vi "ProjectOpenReferences.vi"(0 "Project File Path":path, 5 "Gateway IP Address (\"\": localhost)":string, 11 "error in (no error)":errorcluster, 12 "Username":string, 13 "Password":string) -> (4 "Project File Path out":path, 6 "Gateway IP Address out":string, 15 "error out":errorcluster)   [LabVIEW 2020, in "ni-veristand-steps-runtime-lib.lvlib"]
uses:
  ni-veristand-steps-runtime-lib.lvlib
  controls/VeriStand dotNet References.ctl
  <vilib>/NI VeriStand/Execution/ModelManager/ModelManagerAPI.ctl
  <vilib>/NI VeriStand/Execution/AlarmManager/AlarmManagerAPI.ctl
  <vilib>/NI VeriStand/Execution/ChannelFaultManager/ChannelFaultAPI.ctl
  <vilib>/NI VeriStand/Execution/Workspace/WorkspaceAPI.ctl
  <vilib>/NI VeriStand/Execution/Project/Project Ref.ctl
  <vilib>/NI VeriStand/Execution/Workspace/NI_VS Workspace ExecutionAPI.lvlib
  <vilib>/NI VeriStand/Execution/ChannelFaultManager/NI_VS ChannelFault ExecutionAPI.lvlib
  <vilib>/NI VeriStand/Execution/ModelManager/NI_VS ModelManager ExecutionAPI.lvlib
  NationalInstruments.VeriStand.ClientAPI
  <vilib>/NI VeriStand/Execution/Project/NI_VS Project ExecutionAPI.lvlib
  <vilib>/NI VeriStand/Execution/AlarmManager/NI_VS AlarmManager ExecutionAPI.lvlib
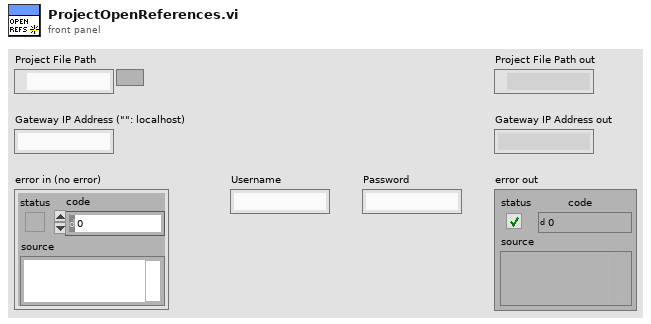
[diagram p1: front panel]
types:
  T1 = typedef "ni-veristand-steps-runtime-lib.lvlib/VeriStand dotNet References.ctl" = cluster{"ModelManager":T2, "AlarmManager":T3, "ChannelFault":T4, "WorkspaceManager":T5, "Project Ref":T6}
  T2 = typedef "NI_VS ModelManager ExecutionAPI.lvlib/ModelManagerAPI.ctl" = refnum<k24>
  T3 = typedef "NI_VS AlarmManager ExecutionAPI.lvlib/AlarmManagerAPI.ctl" = refnum<k24>
  T4 = typedef "NI_VS ChannelFault ExecutionAPI.lvlib/ChannelFaultAPI.ctl" = refnum<k24>
  T5 = typedef "NI_VS Workspace ExecutionAPI.lvlib/WorkspaceAPI.ctl" = refnum<k24>
  T6 = typedef "NI_VS Project ExecutionAPI.lvlib/Project Ref.ctl" = refnum<k24>
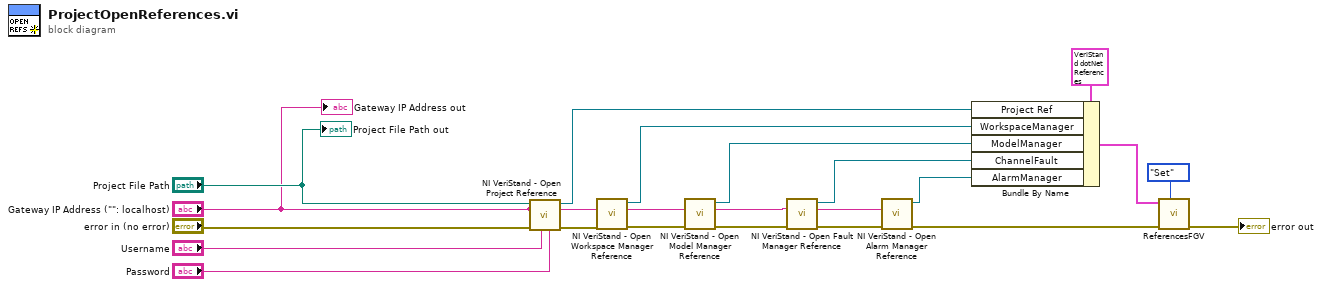
[diagram p0: block diagram]
diagram:
  n1 = call <vilib>:"NI VeriStand - Open Project Reference.vi"("Password"="Password", "Username"="Username", "error in (no error)"="error in (no error)", "Gateway IP Address (\"\": localhost)"="Gateway IP Address (\"\": localhost)", "Project File Path"="Project File Path") -> ("error out"=w6:errorcluster, "Project Ref"=w5:T6)  [unwired: 5 in]
  n2 = call <vilib>:"NI VeriStand - Open Workspace Manager Reference.vi"("error in (no error)"=w6, "Gateway IP Address (\"\": localhost)"="Gateway IP Address (\"\": localhost)") -> ("error out"=w19:errorcluster, "WorkspaceManager"=w12:T5)  [unwired: 8 in]
  n3 = call <vilib>:"NI VeriStand - Open Model Manager Reference.vi"("error in (no error)"=w19, "Gateway IP Address (\"\": localhost)"="Gateway IP Address (\"\": localhost)") -> ("error out"=w18:errorcluster, "ModelManager"=w11:T2)  [unwired: 8 in]
  n4 = call <vilib>:"NI VeriStand - Open Fault Manager Reference.vi"("error in (no error)"=w18, "Gateway IP Address (\"\": localhost)"="Gateway IP Address (\"\": localhost)") -> ("error out"=w3:errorcluster, "ChannelFault"=w10:T4)  [unwired: 8 in]
  n5 = call <vilib>:"NI VeriStand - Open Alarm Manager Reference.vi"("error in (no error)"=w3, "Gateway IP Address (\"\": localhost)"="Gateway IP Address (\"\": localhost)") -> ("error out"=w1:errorcluster, "AlarmManager"=w2:T3)  [unwired: 8 in]
  n6 = Bundle By Name(cluster=T1 {"ModelManager"=refnum, "AlarmManager"=refnum, "ChannelFault"=refnum, "WorkspaceManager"=refnum, "Project Ref"=refnum} ("VeriStand dotNET Refs"), "Project Ref"=w5, "WorkspaceManager"=w12, "ModelManager"=w11, "ChannelFault"=w10, "AlarmManager"=w2) -> (w9:T1)
  n7 = call "ReferencesFGV.vi"("Get/Set"=enum16{"Get", "Set"}."Set", "error in (no error)"=w1, "VeriStand dotNET Refs"=w9) -> ("error out"=→"error out":errorcluster)  [unwired: 7 in, 1 out]
  "Project File Path out" <- "Project File Path"
  "Gateway IP Address out" <- "Gateway IP Address (\"\": localhost)"
